vi "Recover All Persisted Values.vi"(8 "error in (no error)":errorcluster, 11 "Folder Path":path) -> (0 "error out":errorcluster, 2 "Recovered Values":T1[](array[typedef]))   [LabVIEW 2017, in "PersistToDiskTransport.lvclass"]
uses:
  <vilib>/gpm_packages/@cs/transport/Source/Concrete/PersistToDiskTransport/PersistToDiskTransport.lvclass
  <vilib>/gpm_packages/@cs/transport/Source/Concrete/PersistToDiskTransport/Recovered Value.ctl
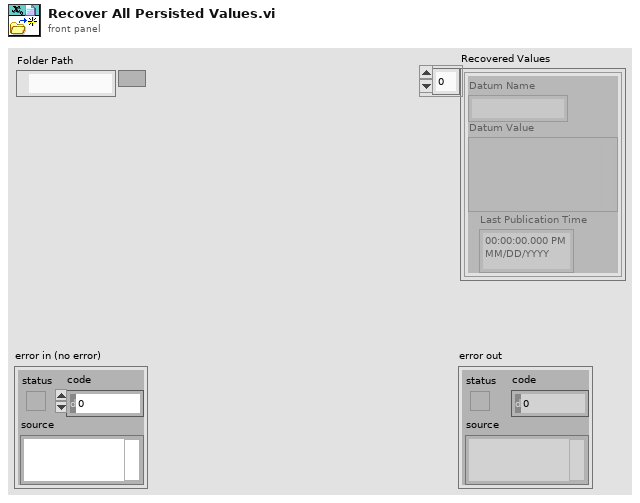
[diagram p1: front panel]
types:
  T1 = typedef "PersistToDiskTransport.lvclass/Recovered Value.ctl" = cluster{"Datum Name":string, "Datum Value":variant, "Last Publication Time":timestamp}
  T2 = cluster{"Datum Name":string, "type string":i16[], "data string":string, "Publication Time":timestamp}
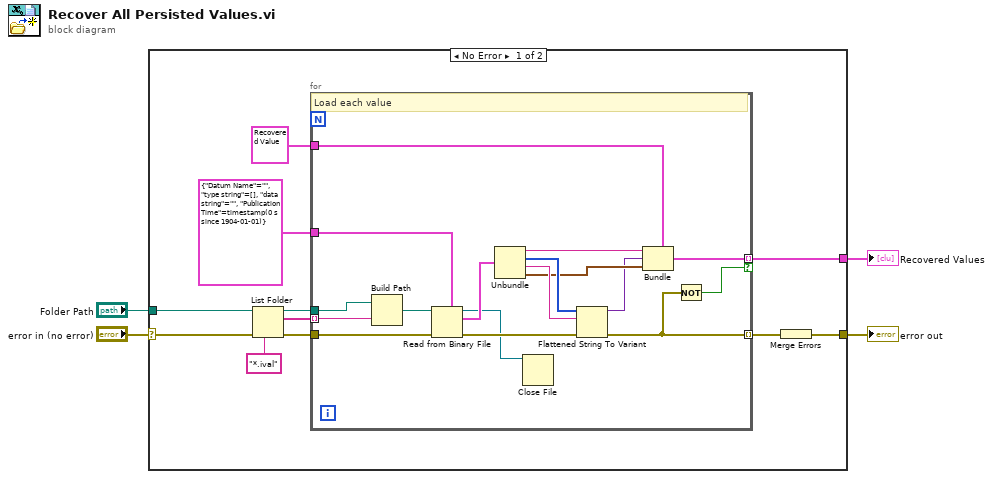
[diagram p0: block diagram]
diagram:
  n1 = case shown="No Error" "error in (no error)" {
    selector: "error in (no error)" -> [w14 w33]
    tunnel: [w7 w33] -> w3
    tunnel: "Folder Path" -> [w15 _]
    tunnel: [w5 _] -> w1
    frame No Error {
      n2 = List Folder(path=w15, pattern="*.ival", error in=w14) -> (path out=w11:path, filenames=w12:string[], error out=w9:errorcluster)  [unwired: 1 in, 1 out]
      n3 = for {
        tunnel: w12 -> [w31] mode=indexing
        tunnel: w11 -> [w32]
        tunnel: T2 {"Datum Name"="", "type string"=[], "data string"="", "Publication Time"=timestamp(0 s since 1904-01-01)} ("cluster") -> [w29]
        tunnel: w9 -> [w28]
        tunnel: [w17] -> w8 mode=indexing
        tunnel: T1 {"Datum Name"="", "Datum Value"=variant, "Last Publication Time"=timestamp(0 s since 1904-01-01)} ("cluster") -> [w20]
        tunnel: [w19] -> w5 mode=indexing if=w16
        # "Load each value"
        n4 = Build Path(base path=w32, name or relative path=w31) -> (appended path=w30:path)
        n5 = Read from Binary File(5:w29, 8:w28, 11:w30) -> (0:w24:errorcluster, 2:w27:T2, 3:w18:refnum<file>)  [unwired: 3 in, 1 out]
        n6 = Unbundle(w27) -> ("Datum Name"=w23:string, "type string"=w26:i16[], "data string"=w25:string, "Publication Time"=w22:timestamp)
        n7 = Close File(refnum=w18) -> ()  [unwired: 1 in, 2 out]
        n8 = Flattened String To Variant(4:w24, 6:w25, 7:w26) -> (0:w17:errorcluster, 3:w21:variant)
        n9 = Bundle(cluster=w20, "Datum Name"=w23, "Datum Value"=w21, "Last Publication Time"=w22) -> (w19:T1)
        n10 = Not(x=w17) -> (.not. x?=w16:bool)
      }
      n11 = Merge Errors(w8) -> (w7:errorcluster)
    }
    frame Error {
    }
  }
  "error out" <- w3
  "Recovered Values" <- w1
